vi "Datasheet Find Run to Use for Plot.vi"(6 "Run Mode":string, 8 "run array":T1[](array[typedef]), 9 "Field Value":string, 10 "Field":string, 11 "Test Type":string) -> (1 "no runs found":bool, 2 "Run to Use":T1, 3 "run used":i32)   [LabVIEW 2011]
uses:
  TDMS/TDMS File.ctl
  TDMS/TDMS Run.ctl
  TDMS/TDMS Channel (Sxx).ctl
  database/Fields/Field Record.ctl
  database/Fields/Field DataTypes.ctl
  database/Fields/Field NextItem.ctl
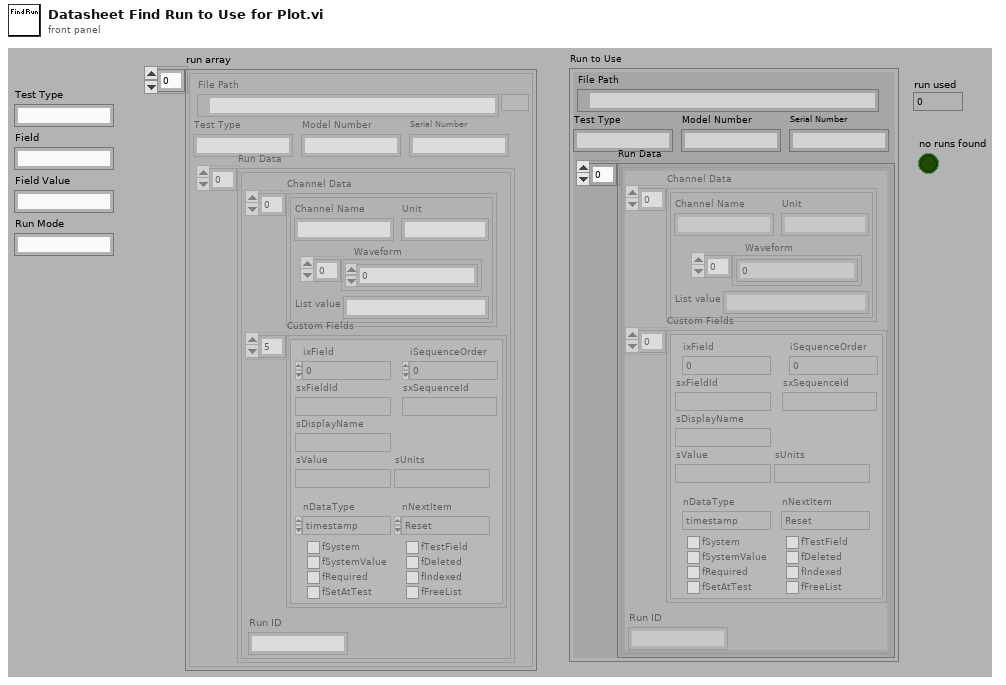
[diagram p1: front panel]
types:
  T1 = typedef "TDMS File.ctl" = cluster{"File Path":path, "Run Data":T2[], "Serial Number":string, "Model Number":string, "Test Type":string}
  T2 = typedef "TDMS Run.ctl" = cluster{"Channel Data":T3[], "Custom Fields":T4[], "Run ID":string}
  T3 = typedef "TDMS Channel (Sxx).ctl" = cluster{"Channel Name":string, "Waveform":dbl[], "Unit":string, "List value":string}
  T4 = typedef "Field Record.ctl" = cluster{"ixField":i32, "iSequenceOrder":i32, "sxFieldId":string, "sxSequenceId":string, "sDisplayName":string, "sValue":string, "sUnits":string, "nDataType":T5, "nNextItem":T6, "fSystem":bool, "fSystemValue":bool, "fRequired":bool, "fSetAtTest":bool, "fTestField":bool, "fDeleted":bool, "fIndexed":bool, "fFreeList":bool}
  T5 = typedef "Field DataTypes.ctl" = enum32{"text", "numeric", "list", "timestamp", "boolean"}
  T6 = typedef "Field NextItem.ctl" = enum32{"Reset", "Retain", "Auto-Increment"}
  T7 = cluster{"File Information":T1, "dimension size":i32}
  T8 = cluster{"File Information":T1, "dimension size":i32}[]
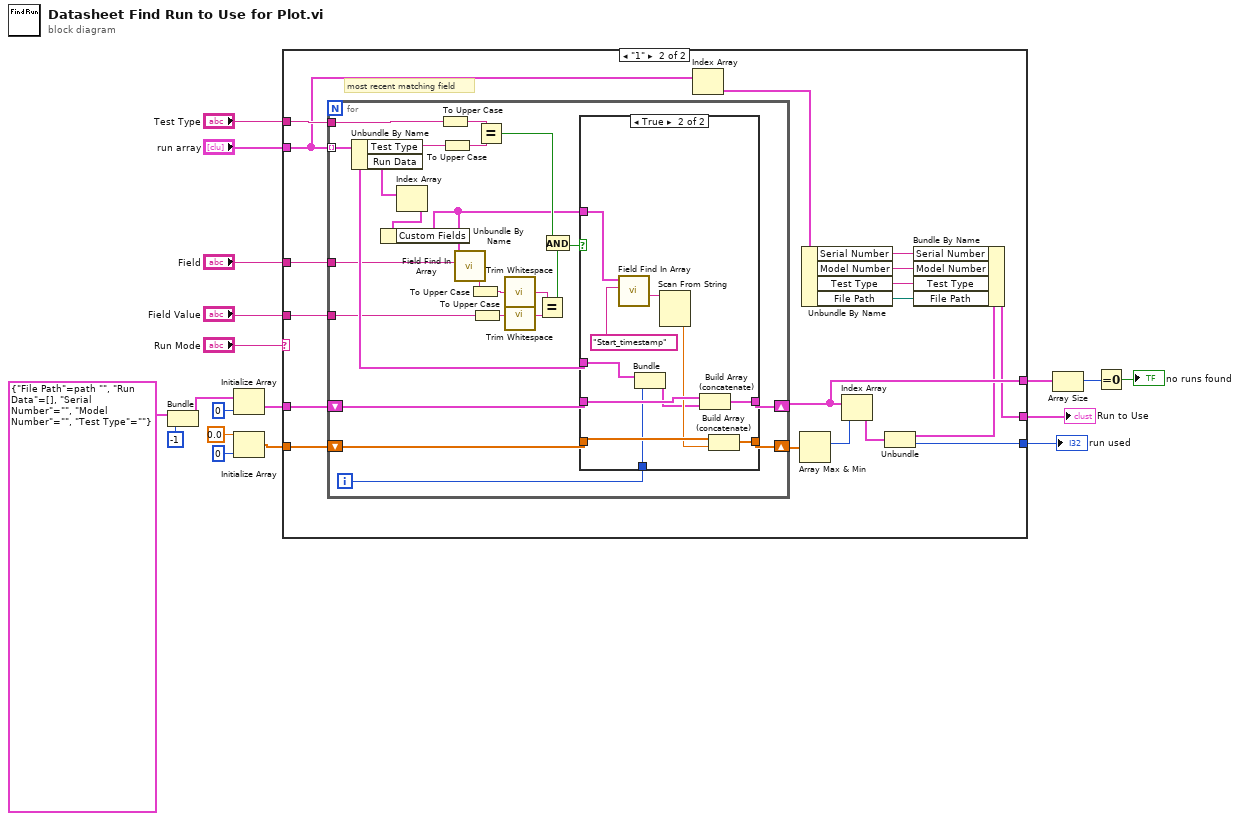
[diagram p0: block diagram]
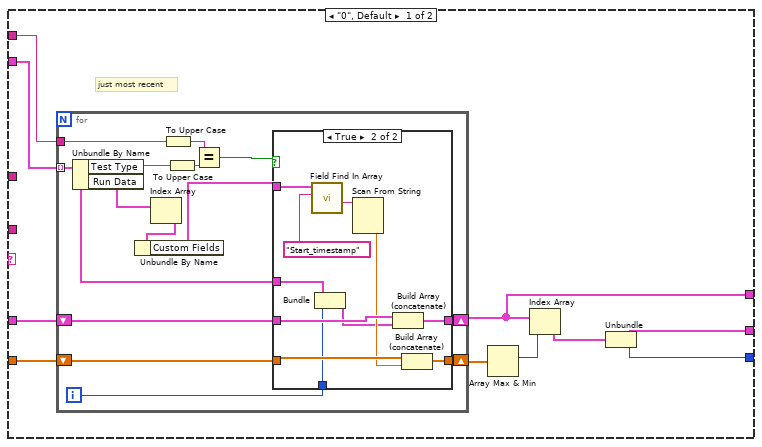
[diagram p2: hidden frame]
diagram:
  n1 = Bundle("File Information"=T1 {"File Path"=path "", "Run Data"=[], "Serial Number"="", "Model Number"="", "Test Type"=""}, "dimension size"=-1) -> (w6:T7)  [unwired: 1 out]
  n2 = Initialize Array(w6, 0 ("dimension size")) -> (w17:T8)
  n3 = Initialize Array(0.0 ("dimension size"), 0 ("dimension size")) -> (w14:dbl[])
  n4 = case shown="\"1\"" "Run Mode" {
    tunnel: w17 -> [w28 w73]
    tunnel: "run array" -> [w27 w63]
    tunnel: "Test Type" -> [w26 w72]
    tunnel: w14 -> [w25 w71]
    tunnel: [w21 w61] -> w12
    tunnel: "Field" -> [_ w68]
    tunnel: "Field Value" -> [_ w67]
    tunnel: [w20 w65] -> w4
    tunnel: [w19 w64] -> w3
    frame "0", Default {
      # "just most recent"
      n5 = for {
        shift-right: [w36] -> w19
        shift-left: w28 -> [w37]
        tunnel: w27 -> [w33] mode=indexing
        tunnel: w26 -> [w41]
        shift-right: [w35] -> w24
        shift-left: w25 -> [w34]
        i -> [w29]
        n6 = Unbundle By Name(w33) -> ("Test Type"=w42:string, "Run Data"=w32:T2[])
        n7 = Index Array(array=w32) -> (element=w31:T2)  [unwired: 1 in]
        n8 = Unbundle By Name(w31) -> ("Custom Fields"=w30:T4[])
        n9 = To Upper Case(1:w41) -> (0:w40:string)
        n10 = To Upper Case(1:w42) -> (0:w39:string)
        n11 = Equal?(x=w40, y=w39) -> (x = y?=w38:bool)
        n12 = case shown="True" w38 {
          tunnel: [w44 w53] -> w36
          tunnel: w37 -> [w44 w52]
          tunnel: [w43 w54] -> w35
          tunnel: w34 -> [w43 w55]
          tunnel: w33 -> [_ w47]
          tunnel: w30 -> [_ w48]
          tunnel: w29 -> [_ w45]
          frame False {
          }
          frame True {
            n13 = call "Field Find In Array.vi"("FieldID or Display Name(\"\")"="Start_timestamp" ("FieldID or Display Name(\"\")"), "Field Array"=w48) -> ("sValue"=w51:string)  [unwired: 1 in, 8 out]
            n14 = Bundle("File Information"=w47, w45) -> (w46:cluster{"File Information":T1, i32})  [unwired: 1 out]
            n15 = Scan From String(input string=w51) -> (output 1=w49:dbl)  [unwired: 3 in, 4 out]
            n16 = Build Array (concatenate)(w52, w46) -> (w53:T8)
            n17 = Build Array (concatenate)(w55, w49) -> (w54:dbl[])
          }
        }
      }
      n18 = Array Max & Min(array=w24) -> (max index (indices)=w23:i32)  [unwired: 3 out]
      n19 = Index Array(array=w19, index=w23) -> (element=w22:T7)
      n20 = Unbundle(w22) -> ("File Information"=w21:T1, "dimension size"=w20:i32)
    }
    frame "1" {
      # "most recent matching field"
      n21 = for {
        shift-right: [w91] -> w64
        shift-left: w73 -> [w92]
        tunnel: w63 -> [w88] mode=indexing
        tunnel: w72 -> [w95]
        shift-right: [w90] -> w70
        shift-left: w71 -> [w89]
        tunnel: w68 -> [w87]
        tunnel: w67 -> [w80]
        i -> [w76]
        n22 = Unbundle By Name(w88) -> ("Test Type"=w96:string, "Run Data"=w78:T2[])
        n23 = Index Array(array=w78) -> (element=w79:T2)  [unwired: 1 in]
        n24 = Unbundle By Name(w79) -> ("Custom Fields"=w77:T4[])
        n25 = To Upper Case(1:w95) -> (0:w94:string)
        n26 = To Upper Case(1:w96) -> (0:w93:string)
        n27 = call "Field Find In Array.vi"("FieldID or Display Name(\"\")"=w87, "Field Array"=w77) -> ("sValue"=w81:string)  [unwired: 1 in, 8 out]
        n28 = To Upper Case(1:w81) -> (0:w84:string)
        n29 = To Upper Case(1:w80) -> (0:w85:string)
        n30 = Equal?(x=w94, y=w93) -> (x = y?=w86:bool)
        n31 = call <vilib>:"Trim Whitespace.vi"("string"=w84) -> ("trimmed string"=w75:string)  [unwired: 1 in]
        n32 = call <vilib>:"Trim Whitespace.vi"("string"=w85) -> ("trimmed string"=w74:string)  [unwired: 1 in]
        n33 = Equal?(x=w75, y=w74) -> (x = y?=w83:bool)
        n34 = And(x=w86, y=w83) -> (x .and. y?=w82:bool)
        n35 = case shown="True" w82 {
          tunnel: [w98 w107] -> w91
          tunnel: w92 -> [w98 w106]
          tunnel: [w97 w108] -> w90
          tunnel: w89 -> [w97 w109]
          tunnel: w88 -> [_ w100]
          tunnel: w77 -> [_ w104]
          tunnel: w76 -> [_ w101]
          frame False {
          }
          frame True {
            n36 = call "Field Find In Array.vi"("FieldID or Display Name(\"\")"="Start_timestamp" ("FieldID or Display Name(\"\")"), "Field Array"=w104) -> ("sValue"=w105:string)  [unwired: 1 in, 8 out]
            n37 = Bundle("File Information"=w100, w101) -> (w99:cluster{"File Information":T1, i32})  [unwired: 1 out]
            n38 = Scan From String(input string=w105) -> (output 1=w102:dbl)  [unwired: 3 in, 4 out]
            n39 = Build Array (concatenate)(w106, w99) -> (w107:T8)
            n40 = Build Array (concatenate)(w109, w102) -> (w108:dbl[])
          }
        }
      }
      n41 = Index Array(array=w63) -> (element=w60:T1)  [unwired: 1 in]
      n42 = Array Max & Min(array=w70) -> (max index (indices)=w69:i32)  [unwired: 3 out]
      n43 = Unbundle By Name(w60) -> ("Serial Number"=w59:string, "Model Number"=w58:string, "Test Type"=w57:string, "File Path"=w56:path)
      n44 = Index Array(array=w64, index=w69) -> (element=w66:T7)
      n45 = Unbundle(w66) -> ("File Information"=w62:T1, "dimension size"=w65:i32)
      n46 = Bundle By Name(cluster=w62, "Serial Number"=w59, "Model Number"=w58, "Test Type"=w57, "File Path"=w56) -> (w61:T1)
    }
  }
  "Run to Use" <- w12
  "run used" <- w4
  n47 = Array Size(array=w3) -> (size(s)=w2:i32)
  n48 = Equal To 0?(x=w2) -> (x = 0?=→"no runs found":bool)
